vi "MS Operation IOP Ctrl v2.vi"(6 "PID Cluster":T3={"L1 to L4 PID Cluster"={"L1 PID Gains"={"Kp"=0.005, "Kd"=0.5, "Ki"=0.0005}, "L2 PID Gains"={"Kp"=0.01, "Kd"=1.0, "Ki"=0.005}, "L3 PID Gains"={"Kp"=0.05, "Kd"=1.0, "Ki"=0.0005}, "L4 PID Gains"={"Kp"=0.1, "Kd"=0.1, "Ki"=0.0005}}, "Stage PID Cluster"={"Stage Z PID"={"Kp"=0.0005, "Kd"=0.001, "Ki"=0.0}, "Stage Y PID"={"Kp"=0.0003, "Kd"=0.01, "Ki"=0.0}, "Stage X PID"={"Kp"=0.0003, "Kd"=0.01, "Ki"=0.0}}, "OCT Z PID Gains"={"Kp"=0.0003, "Kd"=0.0001, "Ki"=0.01}}, 8 "error in":errorcluster, 9 "Offset Home 2 RCM":dbl[](array[numeric])=[0.0, 0.0, 0.0, 0.0], 10 "Prev Posit Cluster":T2={"Prev L1 to L4 Posit"=[-0.5319, -0.035669172703475985, -2.0566170657346783, 0.9099264705882353], "Prev Stage Posit"=[6.002553885707208, 5.996566124542428, 5.995469940427586], "Prev OCT Z Posit"=-0.0}, 11 "FPGA VI Reference In":refnum<k20>) -> (0 "error out":errorcluster, 2 "Last Posit Cluster":T1={"Last L1 to L4 Posit"=[0.0, 0.0, 0.0, 0.0], "Last Stage Posit"=[6.0, 6.0, 6.0], "Last OCT Z Posit"=0.0}, 3 "FPGA VI Reference Out":refnum<k20>)   [LabVIEW 2016]
uses:
  <vilib>/Platform/TimedLoop/XDataNode/timing_clust.ctl
  <vilib>/Platform/TimedLoop/XDataNode/nitl_modes.ctl
  <vilib>/Platform/TimedLoop/XDataNode/wakeup.ctl
  Global Variables.vi
  <vilib>/Utility/error.llb/Error Cluster From Error Code.vi
  <vilib>/rvi/errors/niLvFpgaAdjustHostInterfaceError.vi
  <vilib>/platform/TimedLoop/XDataNode/XDataNode.xnode
  <vilib>/rvi/interface/nirviReadWriteControl/nirviReadWriteControl.xnode
  FPGA Bitfiles/PhantomControlPI_FPGATarget_QuadCtr2_E2412E44.lvbitx
  IRISS_FPGA_IO.vi
  <vilib>/Platform/TimedLoop/XDataNode/XDNodeRunTimeDep.lvlib
  Library/KevinLibraryAll/labview/KevLib01.lvlib
  Library/KevinLibraryAll/labview2011/kevLib2011.lvlib
  NiFpgaLv.dll
panel:
  out "Period [ms]":i64=10
  out "Acc Ctrl Array":dbl[](array[numeric])
  out "L1 to L4 Remote cmd":dbl[](array[numeric])
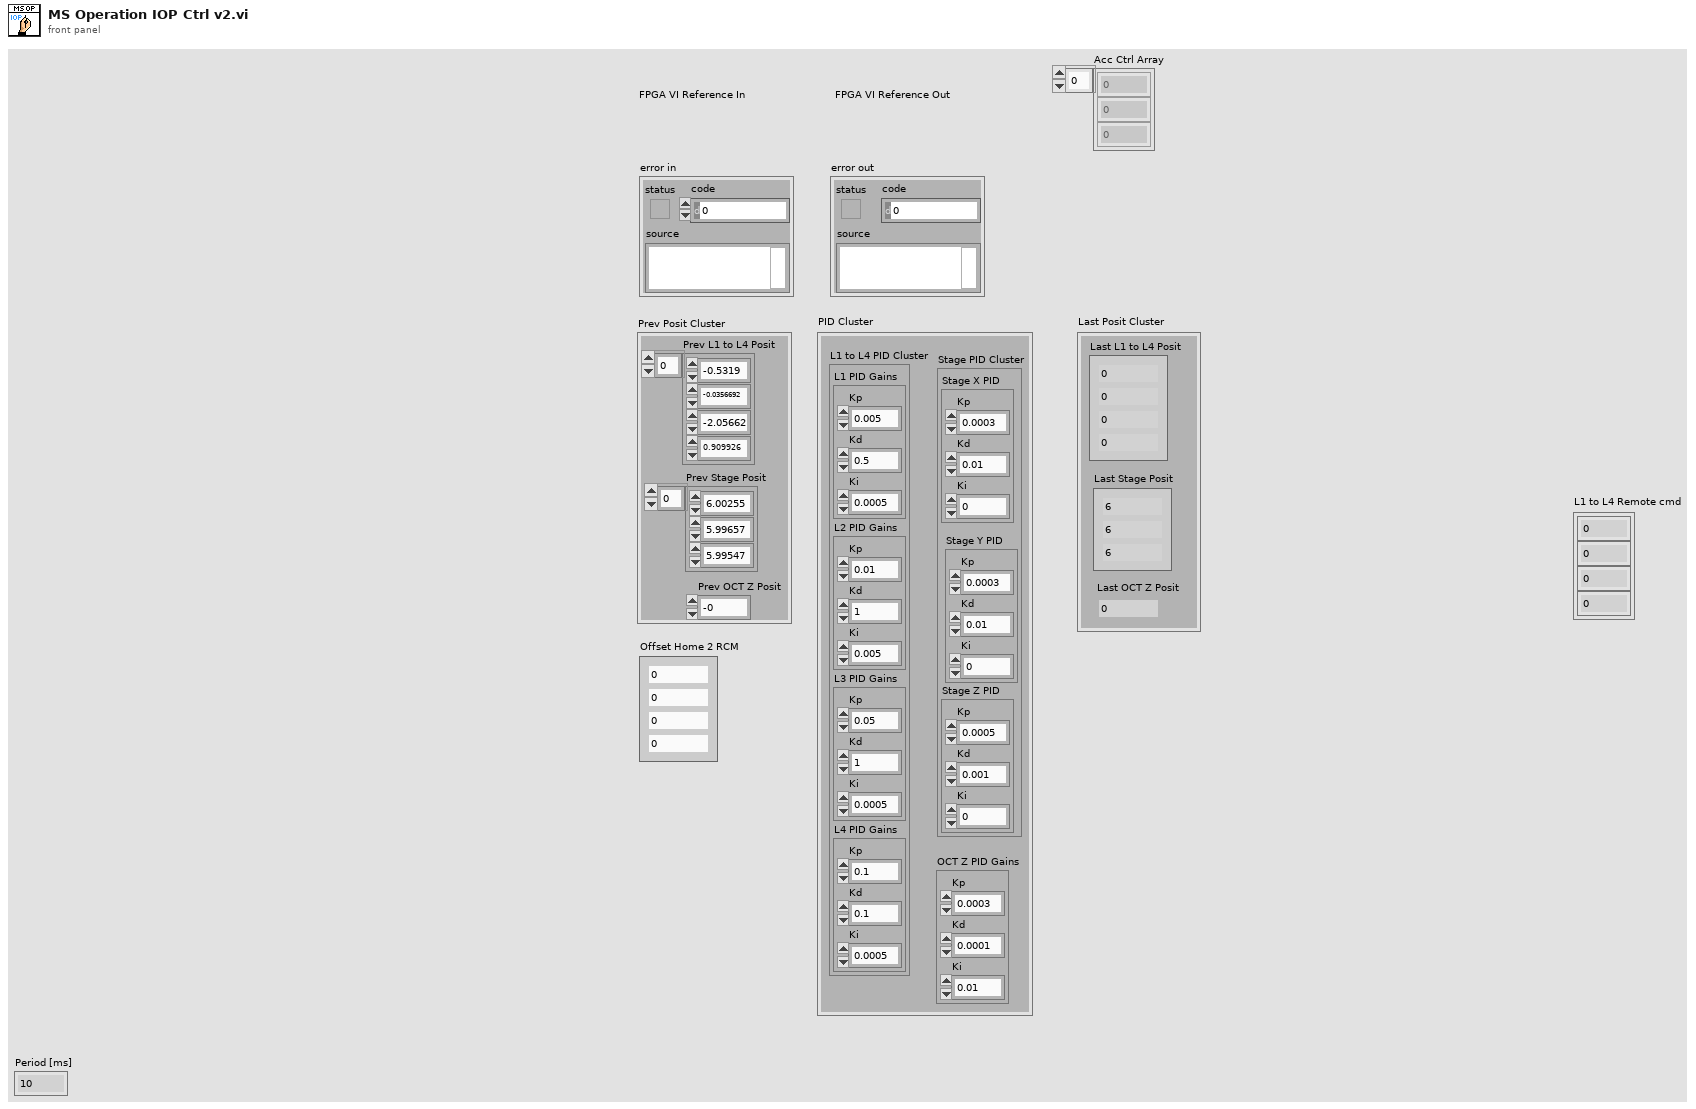
[diagram p1: front panel]
types:
  T1 = cluster{"Last L1 to L4 Posit":dbl[], "Last Stage Posit":dbl[], "Last OCT Z Posit":dbl}
  T2 = cluster{"Prev L1 to L4 Posit":dbl[], "Prev Stage Posit":dbl[], "Prev OCT Z Posit":dbl}
  T3 = cluster{"L1 to L4 PID Cluster":cluster{"L1 PID Gains":cluster{"Kp":dbl, "Kd":dbl, "Ki":dbl}, "L2 PID Gains":cluster{"Kp":dbl, "Kd":dbl, "Ki":dbl}, "L3 PID Gains":cluster{"Kp":dbl, "Kd":dbl, "Ki":dbl}, "L4 PID Gains":cluster{"Kp":dbl, "Kd":dbl, "Ki":dbl}}, "Stage PID Cluster":cluster{"Stage Z PID":cluster{"Kp":dbl, "Kd":dbl, "Ki":dbl}, "Stage Y PID":cluster{"Kp":dbl, "Kd":dbl, "Ki":dbl}, "Stage X PID":cluster{"Kp":dbl, "Kd":dbl, "Ki":dbl}}, "OCT Z PID Gains":cluster{"Kp":dbl, "Kd":dbl, "Ki":dbl}}
  T4 = typedef "XDNodeRunTimeDep.lvlib/timing_clust.ctl" = cluster{"Expected End [f-1]":u64, "Actual End [f-1]":u64, "Finished Late? [f-1]":bool, "Expected End [i-1]":u64, "Actual End [i-1]":u64, "Finished Late? [i-1]":bool, "Expected Start [i]":u64, "Actual Start [i]":u64, "Expected Start [f]":u64, "Actual Start [f]":u64, "Source Name":string, "Structure Name":string, "Period":i64, "Deadline":i64, "Offset":i64, "Start":i64, "Priority":i32, "Timeout":i32, "Mode":T5, "Wakeup Reason":T6, "Error":errorcluster, "Source Type":string, "Secondary Source Type":string, "Global End Time":u64, "Global Start Time":u64, "Frame Duration":u64, "Iteration Duration":u64, "Assigned CPU":i32, "I/O Scan Engine Mode":u32}
  T5 = typedef "XDNodeRunTimeDep.lvlib/nitl_modes.ctl" = enum32{"No Change", "Process missed periods, maintain original phase", "Discard missed periods, maintain original phase", "Process missed periods, ignore original phase", "Discard missed periods, ignore original phase"}
  T6 = typedef "XDNodeRunTimeDep.lvlib/wakeup.ctl" = enum32{"Normal", "Aborted", "Asynchronous wakeup", "Timing source error", "Timed loop error", "Timeout"}
  T7 = cluster{"L1 PID Gains":cluster{"Kp":dbl, "Kd":dbl, "Ki":dbl}, "L2 PID Gains":cluster{"Kp":dbl, "Kd":dbl, "Ki":dbl}, "L3 PID Gains":cluster{"Kp":dbl, "Kd":dbl, "Ki":dbl}, "L4 PID Gains":cluster{"Kp":dbl, "Kd":dbl, "Ki":dbl}}
  T8 = cluster{"Stage Z PID":cluster{"Kp":dbl, "Kd":dbl, "Ki":dbl}, "Stage Y PID":cluster{"Kp":dbl, "Kd":dbl, "Ki":dbl}, "Stage X PID":cluster{"Kp":dbl, "Kd":dbl, "Ki":dbl}}
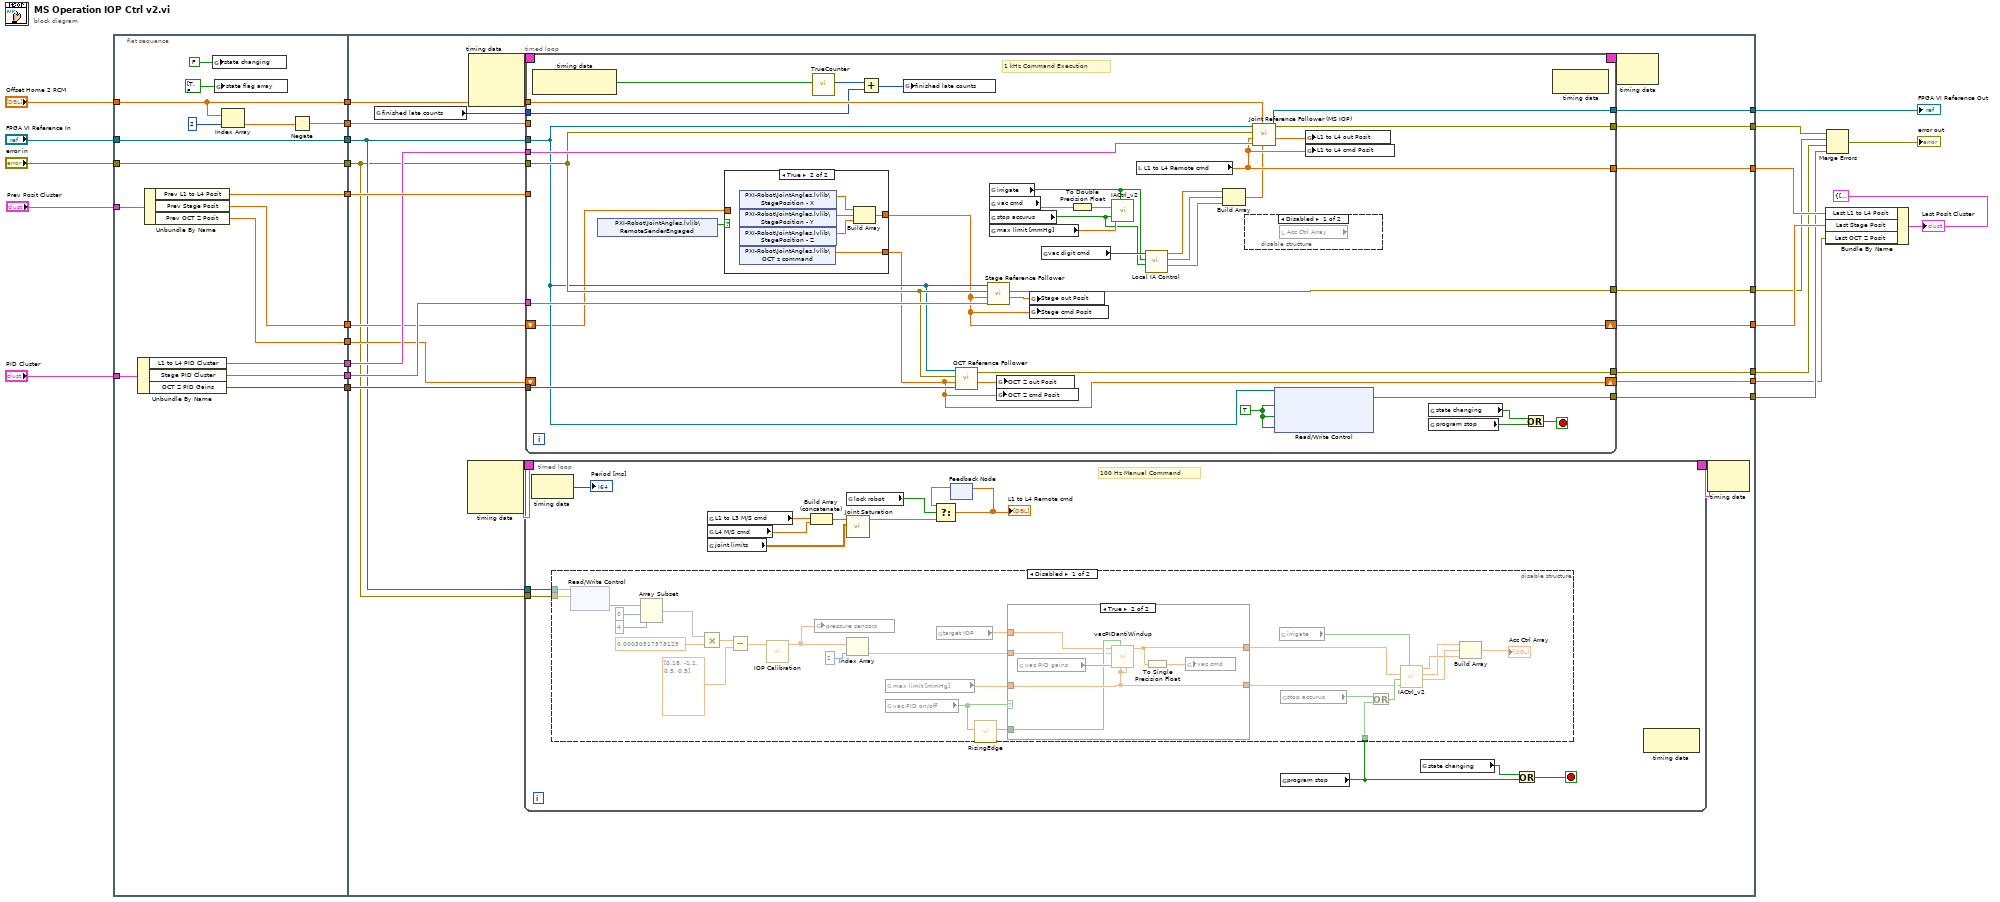
[diagram p0: block diagram]
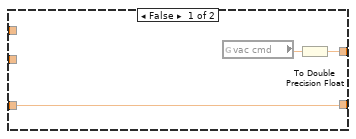
[diagram p2: hidden frame]
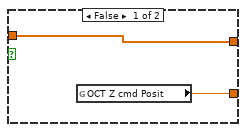
[diagram p5: hidden frame]
diagram:
  n1 = flat-sequence {
    tunnel: [w40] -> w26
    tunnel: "FPGA VI Reference In" -> [w40]
    tunnel: [w39] -> w24
    tunnel: "error in" -> [w39]
    tunnel: [w34] -> w22
    tunnel: "Offset Home 2 RCM" -> [w34]
    tunnel: "Prev Posit Cluster" -> [w29]
    tunnel: [w38] -> w19
    tunnel: "PID Cluster" -> [w37]
    tunnel: [w36] -> w17
    tunnel: [w32] -> w16
    tunnel: [w31] -> w4
    tunnel: [w30] -> w3
    tunnel: [w28] -> w2
    tunnel: [w27] -> w1
    tunnel: w26 -> [w44]
    tunnel: w24 -> [w43]
    tunnel: w22 -> [w61]
    tunnel: w19 -> [w60]
    tunnel: w17 -> [w59]
    tunnel: w16 -> [w58]
    tunnel: [w57] -> w6
    tunnel: [w56] -> w12
    tunnel: [w55] -> w13
    tunnel: [w45] -> w10
    tunnel: [w46] -> w9
    tunnel: [w54] -> w7
    tunnel: [w53] -> w8
    tunnel: [w47] -> w5
    tunnel: w4 -> [w52]
    tunnel: w3 -> [w51]
    tunnel: w2 -> [w49]
    tunnel: w1 -> [w48]
    frame #0 {
      n2 = Unbundle By Name(w37) -> ("L1 to L4 PID Cluster"=w36:T7, "Stage PID Cluster"=w31:T8, "OCT Z PID Gains"=w30:cluster{"Kp":dbl, "Kd":dbl, "Ki":dbl})
      n3 = Unbundle By Name(w29) -> ("Prev L1 to L4 Posit"=w38:dbl[], "Prev Stage Posit"=w28:dbl[], "Prev OCT Z Posit"=w27:dbl)
      n4 = global write "Global Variables.vi" "state changing"(FALSE ("state changing")) -> ()
      n5 = global write "Global Variables.vi" "state flag array"(bool[] [TRUE, FALSE, FALSE, FALSE, FALSE, FALSE, FALSE, FALSE, FALSE] ("state flag array")) -> ()
      n6 = Index Array(array=w34, index=2) -> (element=w33:dbl)
      n7 = Negate(x=w33) -> (-x=w32:dbl)
    }
    frame #1 {
      n8 = global read "Global Variables.vi" "finished late counts"() -> (w50:u16)
      n9 = node-c288() -> (w63:T4)  [unwired: 3 in]
      n10 = node-c288() -> (w65:T4)  [unwired: 3 in]
      n11 = timed-loop {
        timing: w63 -> [_]
        timing-out: [_] -> w62
        tunnel: w44 -> [w74]
        tunnel: w43 -> [w73]
        stop <- w79 stop-if-true
        # "100 Hz Manual Command"
        n12 = node-c288() -> (→"Period [ms]":i64)  [unwired: 1 in]
        n13 = global read "Global Variables.vi" "L1 to L3 M/S cmd"() -> (w70:dbl[])
        n14 = global read "Global Variables.vi" "L4 M/S cmd"() -> (w69:dbl)
        n15 = global read "Global Variables.vi" "joint limits"() -> (w67:dbl[][])
        n16 = Build Array (concatenate)(w70, w69) -> (w68:dbl[])
        n17 = global read "Global Variables.vi" "lock robot"() -> (w77:bool)
        n18 = call "Joint Saturation.vi"("Joint Bounds [Deg/mm]"=w67, "Ref Array [Deg/mm]"=w68) -> ("Sat Ref Array [Deg/mm]"=w66:dbl[])  [unwired: 9 in]
        n19 = feedback #1() -> (w76:dbl[])  [unwired: 1 in]
        n20 = Select(t=w76, s=w77, f=w66) -> (s? t:f=w75:dbl[])
        "L1 to L4 Remote cmd" <- w75
        n21 = feedback-in #1(w75) -> ()
        n22 = global read "Global Variables.vi" "program stop"() -> (w72:bool)
        n23 = disable-structure shown="Disabled" {
          disable-tunnel: w74 -> [w105 _]
          disable-tunnel: w73 -> [w104 _]
          disable-tunnel: w72 -> [w100 _]
          frame Disabled {
            n24 = xnode "Read/Write Control"("FPGA VI Reference In"=w105, "error in"=w104) -> ("AI"=w87:i16[])  [unwired: 2 out]
            n25 = Array Subset(array=w87, index=0, length=4) -> (w92:i16[])
            n26 = Multiply(x=w92, y=0.00030517578125) -> (x*y=w93:dbl[])
            n27 = Subtract(x=w93, y=dbl[] [0.18, -1.1, 0.5, 0.5]) -> (x-y=w88:dbl[])
            n28 = call "IOP Calibration.vi"("IOP Input [V]"=w88) -> ("IOP Output [mmHg]"=w82:dbl[])  [unwired: 10 in]
            n29 = global write "Global Variables.vi" "pressure sensors"(w82) -> ()
            n30 = Index Array(array=w82, index=2) -> (element=w85:dbl)
            n31 = global read "Global Variables.vi" "max limit [mmHg]"() -> (w83:dbl)
            n32 = global read "Global Variables.vi" "vac PID on/off"() -> (w81:bool)
            n33 = global read "Global Variables.vi" "target IOP"() -> (w84:sgl)
            n34 = call "RisingEdge.vi"("Signal In"=w81) -> ("Rising Edge"=w80:bool)  [unwired: 10 in]
            n35 = case shown="True" w81 {
              tunnel: w85 -> [_ w110]
              tunnel: w84 -> [_ w111]
              tunnel: [w107 w115] -> w95
              tunnel: w83 -> [w109 w113]
              tunnel: [w109 w113] -> w99
              tunnel: w80 -> [_ w112]
              frame False {
                n36 = global read "Global Variables.vi" "vac cmd"() -> (w108:sgl)
                n37 = To Double Precision Float(number=w108) -> (double precision float=w107:dbl)
              }
              frame True {
                n38 = global read "Global Variables.vi" "vac PID gains"() -> (w114:cluster{"Kp":dbl, "Kd":dbl, "Ki":dbl, "Ts":dbl})
                n39 = call "vacPIDantiWindup.vi"("Saturation U"=w113, "Saturation M"=w113, "Reset"=w112, "PID Gains"=w114, "Feedback"=w110, "Reference"=w111) -> ("Control"=w115:dbl)  [unwired: 5 in]
                n40 = To Single Precision Float(number=w115) -> (single precision float=w116:sgl)
                n41 = global write "Global Variables.vi" "vac cmd"(w116) -> ()
              }
            }
            n42 = global read "Global Variables.vi" "irrigate"() -> (w98:bool)
            n43 = global read "Global Variables.vi" "stop accurus"() -> (w106:bool)
            n44 = Or(x=w106, y=w100) -> (x .or. y?=w101:bool)
            n45 = call "IACtrl_v2.vi"("Irrigate?"=w98, "Max Limit [mmHg]"=w99, "E-Stop Vacuum"=w101, "Vacuum Force [mmHg]"=w95) -> ("Accurus ChB Vout"=w96:dbl, "Accurus ChA Vout"=w97:dbl, "Accurus Engaged Vout"=w103:dbl)  [unwired: 4 in, 1 out]
            n46 = Build Array(w97, w96, w103) -> (→"Acc Ctrl Array":dbl[])
          }
          frame Enabled {
          }
        }
        n47 = global read "Global Variables.vi" "state changing"() -> (w78:bool)
        n48 = Or(x=w78, y=w72) -> (x .or. y?=w79:bool)
        n49 = node-c288() -> ()  [unwired: 1 in, 1 out]
      }
      n50 = timed-loop {
        timing: w65 -> [_]
        timing-out: [_] -> w64
        tunnel: w44 -> [w136]
        tunnel: w43 -> [w142]
        tunnel: w61 -> [w156]
        tunnel: w60 -> [_]
        tunnel: w59 -> [w155]
        tunnel: w58 -> [_]
        tunnel: [w154] -> w57
        tunnel: [w153] -> w56
        tunnel: [w152] -> w55
        tunnel: [w151] -> w54
        tunnel: [w150] -> w53
        tunnel: w52 -> [w148]
        tunnel: w51 -> [w147]
        tunnel: w50 -> [w143]
        shift-right: [w133] -> w46
        shift-left: w49 -> [w134]
        shift-right: [w132] -> w47
        shift-left: w48 -> [_]
        tunnel: [w138] -> w45
        stop <- w158 stop-if-true
        w137 = TRUE ("Conn0/DIO15 Button 4")
        # "1 kHz Command Execution"
        n51 = node-c288() -> (w146:bool)  [unwired: 1 in]
        n52 = shared-variable "PXI-Robot\\JointAngles.lvlib\\RemoteSenderEngaged"() -> (w135:bool)  [unwired: 1 in, 1 out]
        n53 = case shown="True" w135 {
          tunnel: [w160 w165] -> w133
          tunnel: [w159 w161] -> w132
          tunnel: w134 -> [w160 _]
          frame False {
            n54 = global read "Global Variables.vi" "OCT Z cmd Posit"() -> (w159:dbl)
          }
          frame True {
            n55 = shared-variable "PXI-Robot\\JointAngles.lvlib\\StagePosition - X"() -> (w162:dbl)  [unwired: 1 in, 1 out]
            n56 = shared-variable "PXI-Robot\\JointAngles.lvlib\\StagePosition - Y"() -> (w163:dbl)  [unwired: 1 in, 1 out]
            n57 = shared-variable "PXI-Robot\\JointAngles.lvlib\\StagePosition - Z"() -> (w164:dbl)  [unwired: 1 in, 1 out]
            n58 = shared-variable "PXI-Robot\\JointAngles.lvlib\\OCT z command"() -> (w161:dbl)  [unwired: 1 in, 1 out]
            n59 = Build Array(w162, w163, w164) -> (w165:dbl[])
          }
        }
        n60 = call "TrueCounter.vi"("True?"=w146) -> ("True Count"=w144:u16)  [unwired: 10 in]
        n61 = Add(x=w144, y=w143) -> (x+y=w145:u16)
        n62 = global write "Global Variables.vi" "finished late counts"(w145) -> ()
        n63 = call "OCT Reference Follower.vi"("OCT Z PID Gains"=w147, "OCT  Z cmd Posit [mm]"=w132, "error in"=w142, "FPGA VI Reference In"=w136) -> ("OCT  Z out Posit [mm]"=w141:dbl, "error out"=w151:errorcluster)  [unwired: 5 in, 1 out]
        n64 = call "Stage Reference Follower.vi"("Stage PID Cluster"=w148, "Stage cmd Posit [mm]"=w133, "error in"=w142, "FPGA VI Reference In"=w136) -> ("Stage out Posit [mm]"=w140:dbl[], "error out"=w150:errorcluster)  [unwired: 5 in, 1 out]
        n65 = global read "Global Variables.vi" "irrigate"() -> (w123:bool)
        n66 = global read "Global Variables.vi" "vac cmd"() -> (w131:sgl)
        n67 = global read "Global Variables.vi" "stop accurus"() -> (w122:bool)
        n68 = global read "Global Variables.vi" "max limit [mmHg]"() -> (w129:dbl)
        n69 = global write "Global Variables.vi" "OCT Z cmd Posit"(w132) -> ()
        n70 = global write "Global Variables.vi" "OCT Z out Posit"(w141) -> ()
        n71 = global write "Global Variables.vi" "Stage out Posit"(w140) -> ()
        n72 = global write "Global Variables.vi" "Stage cmd Posit"(w133) -> ()
        n73 = global read "Global Variables.vi" "vac digit cmd"() -> (w127:i8)
        n74 = To Double Precision Float(number=w131) -> (double precision float=w130:dbl)
        n75 = call "IACtrl_v2.vi"("Irrigate?"=w123, "Max Limit [mmHg]"=w129, "E-Stop Vacuum"=w122, "Vacuum Force [mmHg]"=w130) -> ()  [unwired: 4 in, 4 out]
        n76 = local read "L1 to L4 Remote cmd"() -> (w138:dbl[])
        n77 = call "Local IA Control.vi"("E-Stop Vacuum"=w122, "Irrigate?"=w123, "8bit integer"=w127) -> ("Accurus Engaged Vout"=w124:dbl, "Accurus ChB Vout"=w125:dbl, "Accurus ChA Vout"=w126:dbl)  [unwired: 6 in]
        n78 = Build Array(w126, w125, w124) -> (w128:dbl[])
        n79 = disable-structure shown="Disabled" {
          frame Disabled {
            n80 = local read "Acc Ctrl Array"() -> ()  [unwired: 1 out]
          }
          frame Enabled {
          }
        }
        n81 = call "Joint Reference Follower (MS IOP).vi"("Acc Ctrl Array"=w128, "Offset Home2RCM [deg/mm]"=w156, "PID Ctrl Cluster"=w155, "Ref Array [deg/mm]"=w138, "error in"=w142, "FPGA VI Reference In"=w136) -> ("Output Posit Array [deg/mm]"=w139:dbl[], "error out"=w153:errorcluster, "FPGA VI Reference Out"=w152:refnum<k20>)  [unwired: 3 in]
        n82 = xnode "Read/Write Control"("FPGA VI Reference In"=w136, "Conn0/DIO12 Button 1"=w137, "Conn0/DIO13 Button 2"=w137, "Conn0/DIO15 Button 4"=w137) -> ("error out"=w154:errorcluster)  [unwired: 1 in, 1 out]
        n83 = global write "Global Variables.vi" "L1 to L4 out Posit"(w139) -> ()
        n84 = global write "Global Variables.vi" "L1 to L4 cmd Posit"(w138) -> ()
        n85 = global read "Global Variables.vi" "state changing"() -> (w157:bool)
        n86 = global read "Global Variables.vi" "program stop"() -> (w149:bool)
        n87 = Or(x=w157, y=w149) -> (x .or. y?=w158:bool)
        n88 = node-c288() -> ()  [unwired: 1 in, 1 out]
      }
      n89 = node-c288(w64) -> ()  [unwired: 1 out]
      n90 = node-c288(w62) -> ()  [unwired: 1 out]
    }
  }
  n91 = Bundle By Name(cluster=T1 {"Last L1 to L4 Posit"=[-0.5607, -0.038216970753724266, -2.0806193533568895, 1.1787683823529411], "Last Stage Posit"=[6.002553885707208, 5.996566124542428, 5.995469940427586], "Last OCT Z Posit"=-0.0} ("Last Posit Cluster 2"), "Last L1 to L4 Posit"=w10, "Last Stage Posit"=w9, "Last OCT Z Posit"=w5) -> (→"Last Posit Cluster":T1)
  n92 = Merge Errors(w12, w8, w7, w6) -> (→"error out":errorcluster)
  "FPGA VI Reference Out" <- w13
